vi "process.vi"(8 "error in":errorcluster, 9 "result allocation":T1, 10 "parameters":T1, 11 "module in":refnum<class "Polynomial Scale runtime.lvclass">) -> (0 "error out":errorcluster, 1 "results":T1, 2 "parameter allocation":T1, 3 "module out":refnum<class "Polynomial Scale runtime.lvclass">)   [LabVIEW 2013, in "Polynomial Scale runtime.lvclass"]
doc: "Provides an interface for information processing by a module at runtime. While this interface performs no operations, a child should provide an override which may process data in any manner necessary."
uses:
  Polynomial Scale runtime.lvclass
  <vilib>/NI/Tag Bus/table/data table.ctl
  <vilib>/NI/DCAF Templates/DCAF Scaling/module/execution/Scaling runtime.lvclass/Scaling runtime.ctl
  Polynomial Scale runtime.lvclass/Polynomial Scale runtime.ctl
  <vilib>/NI/Tag Bus/table/data polymorphs/read one/read Double.vi
  <vilib>/NI/Tag Bus/table/data polymorphs/read one/read Single.vi
  <vilib>/NI/Tag Bus/table/data polymorphs/read one/read I64.vi
  <vilib>/NI/Tag Bus/table/data polymorphs/read one/read I32.vi
  <vilib>/NI/Tag Bus/table/data polymorphs/read one/read I16.vi
  <vilib>/NI/Tag Bus/table/data polymorphs/read one/read I8.vi
  <vilib>/NI/Tag Bus/table/data polymorphs/read one/read U64.vi
  <vilib>/NI/Tag Bus/table/data polymorphs/read one/read U32.vi
  <vilib>/NI/Tag Bus/table/data polymorphs/read one/read U16.vi
  <vilib>/NI/Tag Bus/table/data polymorphs/read one/read U8.vi
  <vilib>/NI/Tag Bus/table/data polymorphs/write one/write Double.vi
  <vilib>/NI/Tag Bus/table/data polymorphs/write one/write Single.vi
  <vilib>/NI/Tag Bus/table/data polymorphs/write one/write I64.vi
  <vilib>/NI/Tag Bus/table/data polymorphs/write one/write I32.vi
  <vilib>/NI/Tag Bus/table/data polymorphs/write one/write I16.vi
  <vilib>/NI/Tag Bus/table/data polymorphs/write one/write I8.vi
  <vilib>/NI/Tag Bus/table/data polymorphs/write one/write U64.vi
  <vilib>/NI/Tag Bus/table/data polymorphs/write one/write U32.vi
  <vilib>/NI/Tag Bus/table/data polymorphs/write one/write U16.vi
  <vilib>/NI/Tag Bus/table/data polymorphs/write one/write U8.vi
  <vilib>/Analysis/polynomials.llb/1D Polynomial Evaluation (DBL).vi
  <vilib>/Analysis/NI_AALPro.lvlib
  <vilib>/NI/Tag Bus/table/data table.lvlib
  <vilib>/NI/DCAF Templates/DCAF Scaling/module/execution/Scaling runtime.lvclass
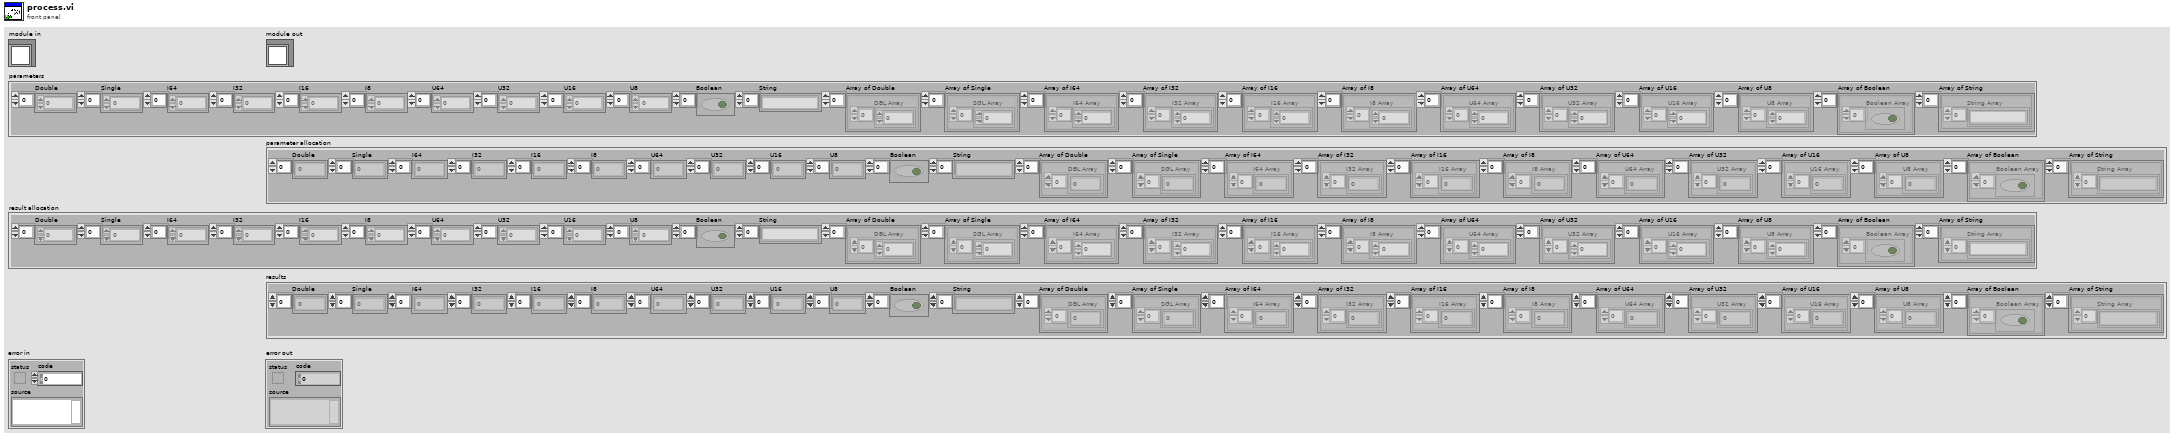
[diagram p1: front panel]
types:
  T1 = typedef "tag bus.lvlib/data table.lvlib/data table.ctl" = cluster{"Double":dbl[], "Single":sgl[], "I64":i64[], "I32":i32[], "I16":i16[], "I8":i8[], "U64":u64[], "U32":u32[], "U16":u16[], "U8":u8[], "Boolean":bool[], "String":string[], "Array of Double":cluster{"DBL Array":dbl[]}[], "Array of Single":cluster{"SGL Array":sgl[]}[], "Array of I64":cluster{"I64 Array":i64[]}[], "Array of I32":cluster{"I32 Array":i32[]}[], "Array of I16":cluster{"I16 Array":i16[]}[], "Array of I8":cluster{"I8 Array":i8[]}[], "Array of U64":cluster{"U64 Array":u64[]}[], "Array of U32":cluster{"U32 Array":u32[]}[], "Array of U16":cluster{"U16 Array":u16[]}[], "Array of U8":cluster{"U8 Array":u8[]}[], "Array of Boolean":cluster{"Boolean Array":bool[]}[], "Array of String":cluster{"String Array":string[]}[]}
  T2 = typedef "tag bus.lvlib/tag descriptor.lvclass/Data Type.ctl" = enum16{"Double", "Single", "I64", "I32", "I16", "I8", "U64", "U32", "U16", "U8", "Boolean", "String", "Array of Double", "Array of Single", "Array of I64", "Array of I32", "Array of I16", "Array of I8", "Array of U64", "Array of U32", "Array of U16", "Array of U8", "Array of Boolean", "Array of String"}
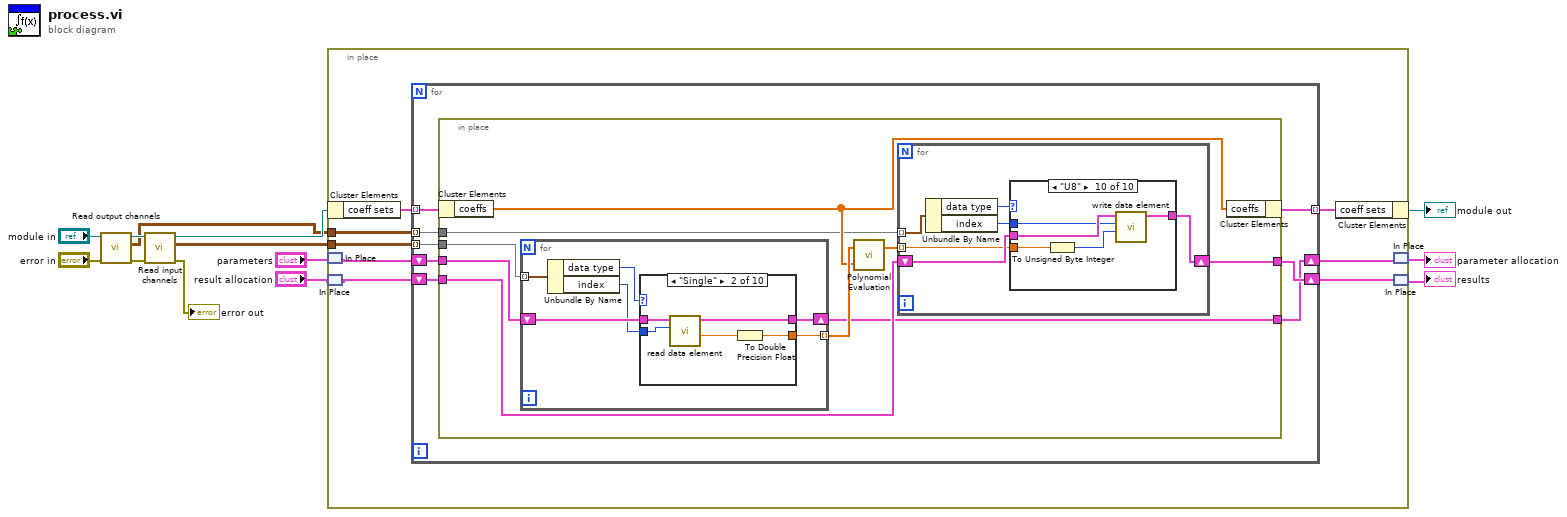
[diagram p0: block diagram]
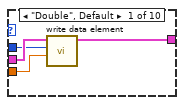
[diagram p2: hidden frame]
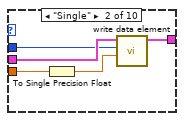
[diagram p3: hidden frame]
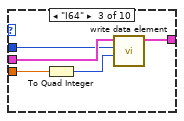
[diagram p4: hidden frame]
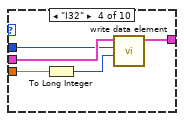
[diagram p5: hidden frame]
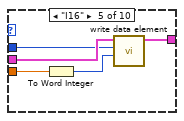
[diagram p6: hidden frame]
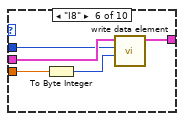
[diagram p7: hidden frame]
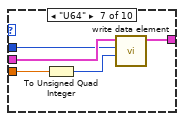
[diagram p8: hidden frame]
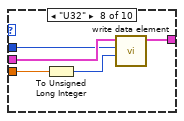
[diagram p9: hidden frame]
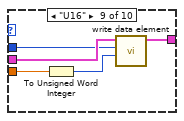
[diagram p10: hidden frame]
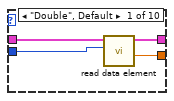
[diagram p11: hidden frame]
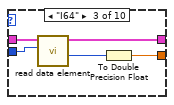
[diagram p12: hidden frame]
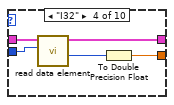
[diagram p13: hidden frame]
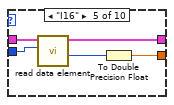
[diagram p14: hidden frame]
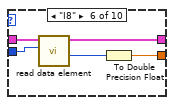
[diagram p15: hidden frame]
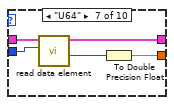
[diagram p16: hidden frame]
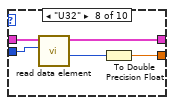
[diagram p17: hidden frame]
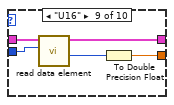
[diagram p18: hidden frame]
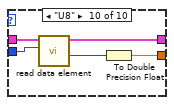
[diagram p19: hidden frame]
diagram:
  n1 = call <vilib>:"Read output channels.vi"("error in (no error)"="error in", "Scaling runtime in"="module in") -> ("error out"=w12:errorcluster, "output channels"=w6:cluster{"data type":T2, "index":i32}[][], "Scaling runtime out"=w13:refnum<class "Polynomial Scale runtime.lvclass">)  [unwired: 7 in]
  n2 = call <vilib>:"Read input channels.vi"("error in (no error)"=w12, "Scaling runtime in"=w13) -> ("error out"=→"error out":errorcluster, "input channels"=w7:cluster{"data type":T2, "index":i32}[][], "Scaling runtime out"=w9:refnum<class "Polynomial Scale runtime.lvclass">)  [unwired: 7 in]
  n3 = in-place {
    in-place-border: w7 -> [w20]
    in-place-border: w6 -> [w19]
    n4 = in-place-cluster #1(w9) -> ("coeff sets"=w21:cluster{"coeffs":dbl[]}[])
    n5 = in-place-match #2("parameters") -> (w17:T1)
    n6 = in-place-match #3("result allocation") -> (w15:T1)
    n7 = for {
      shift-right: [w24] -> w16
      shift-left: w17 -> [w29]
      shift-right: [w25] -> w14
      shift-left: w15 -> [w26]
      tunnel: w21 -> [w23] mode=indexing
      tunnel: w20 -> [w28] mode=indexing
      tunnel: w19 -> [w27] mode=indexing
      tunnel: [w22] -> w18 mode=indexing
      n8 = in-place {
        in-place-border: w29 -> [w37]
        in-place-border: w28 -> [w36]
        in-place-border: w27 -> [w33]
        in-place-border: w26 -> [w32]
        in-place-border: [w31] -> w25
        in-place-border: [w30] -> w24
        n9 = in-place-cluster #4(w23) -> ("coeffs"=w34:dbl[])
        n10 = for {
          shift-right: [w96] -> w30
          shift-left: w37 -> [w97]
          tunnel: w36 -> [w99] mode=indexing
          tunnel: [w95] -> w35 mode=indexing
          n11 = Unbundle By Name(w99) -> ("data type"=w98:T2, "index"=w94:i32)
          n12 = case shown="\"Single\"" w98 {
            tunnel: w97 -> [w103 w108 w113 w118 w123 w128 w133 w138 w143 w148]
            tunnel: [w102 w107 w112 w117 w122 w127 w132 w137 w142 w147] -> w96
            tunnel: [w101 w105 w110 w115 w120 w125 w130 w135 w140 w145] -> w95
            tunnel: w94 -> [w100 w104 w109 w114 w119 w124 w129 w134 w139 w144]
            frame "Double", Default {
              n13 = call-poly <vilib>:"read data element.vi"("index"=w100, "data table in"=w103) -> ("value"=w101:dbl, "data table out"=w102:T1)  [unwired: 8 in]
            }
            frame "Single" {
              n14 = call-poly <vilib>:"read data element.vi"("index"=w104, "data table in"=w108) -> ("value"=w106:sgl, "data table out"=w107:T1)  [unwired: 8 in]
              n15 = To Double Precision Float(number=w106) -> (double precision float=w105:dbl)
            }
            frame "I64" {
              n16 = call-poly <vilib>:"read data element.vi"("index"=w109, "data table in"=w113) -> ("value"=w111:i64, "data table out"=w112:T1)  [unwired: 8 in]
              n17 = To Double Precision Float(number=w111) -> (double precision float=w110:dbl)
            }
            frame "I32" {
              n18 = call-poly <vilib>:"read data element.vi"("index"=w114, "data table in"=w118) -> ("value"=w116:i32, "data table out"=w117:T1)  [unwired: 8 in]
              n19 = To Double Precision Float(number=w116) -> (double precision float=w115:dbl)
            }
            frame "I16" {
              n20 = call-poly <vilib>:"read data element.vi"("index"=w119, "data table in"=w123) -> ("value"=w121:i16, "data table out"=w122:T1)  [unwired: 8 in]
              n21 = To Double Precision Float(number=w121) -> (double precision float=w120:dbl)
            }
            frame "I8" {
              n22 = call-poly <vilib>:"read data element.vi"("index"=w124, "data table in"=w128) -> ("value"=w126:i8, "data table out"=w127:T1)  [unwired: 8 in]
              n23 = To Double Precision Float(number=w126) -> (double precision float=w125:dbl)
            }
            frame "U64" {
              n24 = call-poly <vilib>:"read data element.vi"("index"=w129, "data table in"=w133) -> ("value"=w131:u64, "data table out"=w132:T1)  [unwired: 8 in]
              n25 = To Double Precision Float(number=w131) -> (double precision float=w130:dbl)
            }
            frame "U32" {
              n26 = call-poly <vilib>:"read data element.vi"("index"=w134, "data table in"=w138) -> ("value"=w136:u32, "data table out"=w137:T1)  [unwired: 8 in]
              n27 = To Double Precision Float(number=w136) -> (double precision float=w135:dbl)
            }
            frame "U16" {
              n28 = call-poly <vilib>:"read data element.vi"("index"=w139, "data table in"=w143) -> ("value"=w141:u16, "data table out"=w142:T1)  [unwired: 8 in]
              n29 = To Double Precision Float(number=w141) -> (double precision float=w140:dbl)
            }
            frame "U8" {
              n30 = call-poly <vilib>:"read data element.vi"("index"=w144, "data table in"=w148) -> ("value"=w146:u8, "data table out"=w147:T1)  [unwired: 8 in]
              n31 = To Double Precision Float(number=w146) -> (double precision float=w145:dbl)
            }
          }
        }
        n32 = call-poly <vilib>:"Polynomial Evaluation.vi"("P(x)"=w34, "A"=w35) -> ("P(A)"=w38:dbl[])  [unwired: 1 out]
        n33 = for {
          tunnel: w38 -> [w39] mode=indexing
          tunnel: w33 -> [w44] mode=indexing
          shift-right: [w41] -> w31
          shift-left: w32 -> [w42]
          n34 = Unbundle By Name(w44) -> ("data type"=w43:T2, "index"=w40:i32)
          n35 = case shown="\"U8\"" w43 {
            tunnel: w42 -> [w48 w53 w58 w63 w68 w73 w78 w83 w88 w93]
            tunnel: [w47 w52 w57 w62 w67 w72 w77 w82 w87 w92] -> w41
            tunnel: w40 -> [w46 w51 w56 w61 w66 w71 w76 w81 w86 w91]
            tunnel: w39 -> [w45 w50 w55 w60 w65 w70 w75 w80 w85 w90]
            frame "Double", Default {
              n36 = call-poly <vilib>:"write data element.vi"("value"=w45, "index"=w46, "data table in"=w48) -> ("data table out"=w47:T1)  [unwired: 8 in]
            }
            frame "Single" {
              n37 = To Single Precision Float(number=w50) -> (single precision float=w49:sgl)
              n38 = call-poly <vilib>:"write data element.vi"("value"=w49, "index"=w51, "data table in"=w53) -> ("data table out"=w52:T1)  [unwired: 8 in]
            }
            frame "I64" {
              n39 = To Quad Integer(1:w55) -> (0:w54:i64)
              n40 = call-poly <vilib>:"write data element.vi"("value"=w54, "index"=w56, "data table in"=w58) -> ("data table out"=w57:T1)  [unwired: 8 in]
            }
            frame "I32" {
              n41 = To Long Integer(number=w60) -> (32bit integer=w59:i32)
              n42 = call-poly <vilib>:"write data element.vi"("value"=w59, "index"=w61, "data table in"=w63) -> ("data table out"=w62:T1)  [unwired: 8 in]
            }
            frame "I16" {
              n43 = To Word Integer(number=w65) -> (16bit integer=w64:i16)
              n44 = call-poly <vilib>:"write data element.vi"("value"=w64, "index"=w66, "data table in"=w68) -> ("data table out"=w67:T1)  [unwired: 8 in]
            }
            frame "I8" {
              n45 = To Byte Integer(number=w70) -> (8bit integer=w69:i8)
              n46 = call-poly <vilib>:"write data element.vi"("value"=w69, "index"=w71, "data table in"=w73) -> ("data table out"=w72:T1)  [unwired: 8 in]
            }
            frame "U64" {
              n47 = To Unsigned Quad Integer(1:w75) -> (0:w74:u64)
              n48 = call-poly <vilib>:"write data element.vi"("value"=w74, "index"=w76, "data table in"=w78) -> ("data table out"=w77:T1)  [unwired: 8 in]
            }
            frame "U32" {
              n49 = To Unsigned Long Integer(number=w80) -> (unsigned 32bit integer=w79:u32)
              n50 = call-poly <vilib>:"write data element.vi"("value"=w79, "index"=w81, "data table in"=w83) -> ("data table out"=w82:T1)  [unwired: 8 in]
            }
            frame "U16" {
              n51 = To Unsigned Word Integer(number=w85) -> (unsigned 16bit integer=w84:u16)
              n52 = call-poly <vilib>:"write data element.vi"("value"=w84, "index"=w86, "data table in"=w88) -> ("data table out"=w87:T1)  [unwired: 8 in]
            }
            frame "U8" {
              n53 = To Unsigned Byte Integer(number=w90) -> (unsigned 8bit integer=w89:u8)
              n54 = call-poly <vilib>:"write data element.vi"("value"=w89, "index"=w91, "data table in"=w93) -> ("data table out"=w92:T1)  [unwired: 8 in]
            }
          }
        }
        n55 = in-place-cluster #4("coeffs"=w34) -> (w22:cluster{"coeffs":dbl[]})
      }
    }
    n56 = in-place-cluster #1("coeff sets"=w18) -> (→"module out":refnum<class "Polynomial Scale runtime.lvclass">)
    n57 = in-place-match #2(w16) -> (→"parameter allocation":T1)
    n58 = in-place-match #3(w14) -> (→"results":T1)
  }
